vi "Write Child Unified Actor DVR Map.vi"(10 "Child Unified Actor DVR Map":T1, 11 "Actor in":refnum<class "Actor.lvclass">) -> (3 "Actor out":refnum<class "Actor.lvclass">)   [LabVIEW 2020, in "jettl.lvlib" / "Actor.lvclass"]
uses:
  Actor.lvclass
  Child Unified Actor DVR Map.ctl
  jettl.lvlib
  Unified Actor.ctl
  Msg/Msg.lvclass
  Msg Set.ctl
  Msg Input/Msg Input.lvclass
  Msg Output/Msg Output.lvclass
  Unified Actor Relation.ctl
  Teller.ctl
  Msg.ctl
  Msgs.ctl
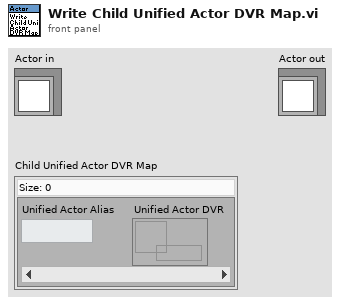
[diagram p1: front panel]
types:
  T1 = typedef "jettl.lvlib/Child Unified Actor DVR Map.ctl" = map{string, refnum<data-value>}
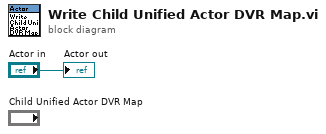
[diagram p0: block diagram]
diagram:
  "Actor out" <- "Actor in"
